vi "pythonDisplayImage.vi"(1 "refresh_time":i32=100, 2 "image reference":refnum<data-value>) -> ()   [LabVIEW 2017]
uses:
  globalUtilities.vi
  dll/wormUtilities/x64/Release/wormUtilities.dll
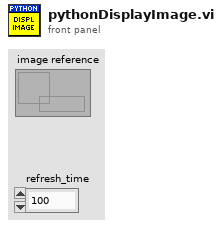
[diagram p1: front panel]
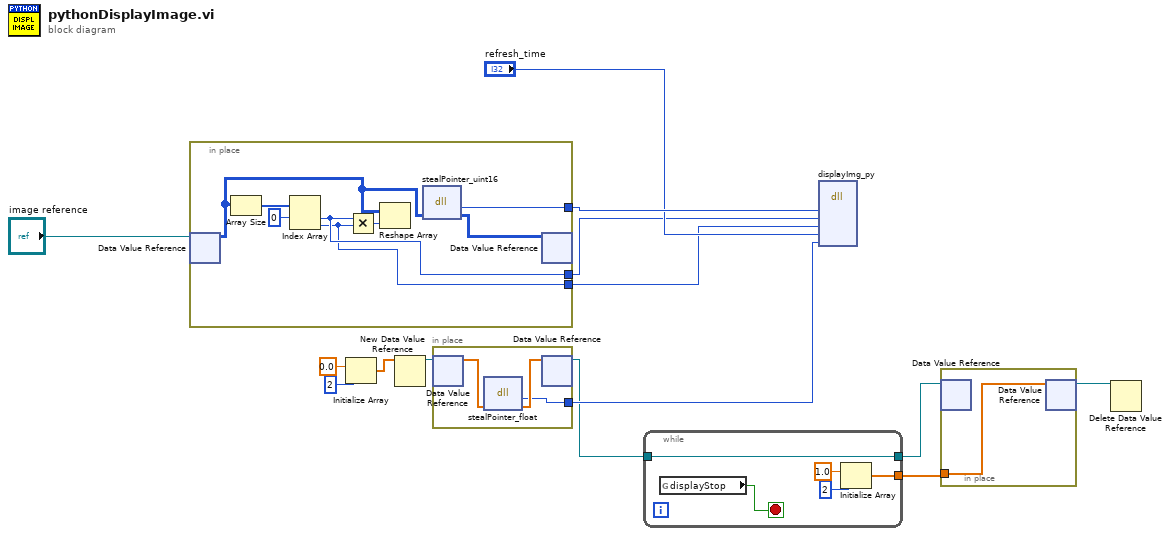
[diagram p0: block diagram]
diagram:
  n1 = in-place {
    in-place-border: [w22] -> w14
    in-place-border: [w18] -> w2
    in-place-border: [w17] -> w1
    n2 = in-place-dvr #1("image reference") -> (w16:u16[][])  [unwired: 1 out]
    n3 = Array Size(array=w16) -> (size(s)=w21:i32[])
    n4 = Index Array(array=w21, index #1=0 ("index")) -> (element #1=w18:i32, element #2=w17:i32)  [unwired: 1 in]
    n5 = Multiply(x=w18, y=w17) -> (x*y=w20:i32)
    n6 = Reshape Array(w16, w20) -> ()  [unwired: 1 out]
    n7 = dll-call lib="C:/Users/francesco/dev/pump-probe/dll/wormUtilities/x64/Release/wormUtilities.dll" fn="stealPointer_uint16"("A"=w16) -> ("return type"=w22:i64, "A"=w15:u16[][])  [unwired: 3 in, 2 out]
    n8 = in-place-dvr #1(w15) -> ()  [unwired: 2 out]
  }
  n9 = Initialize Array(sgl 0.0 ("element"), 2 ("dimension size")) -> (w9:sgl[])
  n10 = New Data Value Reference(data value=w9) -> (data value reference=w12:refnum<data-value>)  [unwired: 1 in, 1 out]
  n11 = in-place {
    in-place-border: [w23] -> w13
    n12 = in-place-dvr #2(w12) -> (w24:sgl[])  [unwired: 1 out]
    n13 = dll-call lib="C:/Users/francesco/dev/pump-probe/dll/wormUtilities/x64/Release/wormUtilities.dll" fn="stealPointer_float"("A"=w24) -> ("return type"=w23:i64, "A"=w25:sgl[])  [unwired: 3 in, 2 out]
    n14 = in-place-dvr #2(w25) -> (w8:refnum<data-value>)  [unwired: 1 out]
  }
  n15 = while {
    tunnel: w8 -> [w29]
    tunnel: [w29] -> w7
    tunnel: [w26] -> w6
    stop <- w30 stop-if-true
    n16 = global read "globalUtilities.vi" "displayStop"() -> (w30:bool)
    n17 = Initialize Array(sgl 1.0 ("element"), 2 ("dimension size")) -> (w26:sgl[])
  }
  n18 = dll-call lib="C:/Users/francesco/dev/pump-probe/dll/wormUtilities/x64/Release/wormUtilities.dll" fn="displayImg_py"("A"=w14, "sizex"=w2, "sizey"=w1, "refresh_time"="refresh_time", "stop"=w13) -> ()  [unwired: 9 in, 2 out]
  n19 = in-place {
    in-place-border: w6 -> [w31]
    n20 = in-place-dvr #3(w7) -> ()  [unwired: 2 out]
    n21 = in-place-dvr #3(w31) -> (w5:refnum<data-value>)  [unwired: 1 out]
  }
  n22 = Delete Data Value Reference(data value reference=w5) -> ()  [unwired: 1 in, 2 out]
